vi "fpga_status.vi"(8 "error in (no error)":errorcluster, 11 "pulse_gen_and_detect_p2p in":refnum<class "pulse_gen_and_detect_p2p.lvclass">) -> (0 "error out":errorcluster, 2 "pulse TX status":T1, 3 "pulse_gen_and_detect_p2p out":refnum<class "pulse_gen_and_detect_p2p.lvclass">)   [LabVIEW 2021, in "pulse_gen_and_detect_p2p.lvclass"]
uses:
  pulse_gen_and_detect_p2p.lvclass
  pulse_gen_and_detect_p2p.lvclass/pulse_gen_and_detect_p2p.ctl
  fpga/vis/pulse detector/PDW interpoter params.ctl
  <vilib>/Utility/error.llb/Error Cluster From Error Code.vi
  <vilib>/rvi/errors/niLvFpgaAdjustHostInterfaceError.vi
  <vilib>/rvi/interface/nirviReadWriteControl/nirviReadWriteControl.xnode
  <vilib>/rvi/interface/nirviMethod/nirviMethod.xnode
  <resource>/objmgr/PeerToPeerStream.rc
  <vilib>/FPGAPlugInAG/Dynamic/niLvFpga_ReadFifo_Dynamic.vi
  <vilib>/rvi/errors/niLvFpgaMergeErrorWithErrorCode.vi
  NiFpgaLv.dll
  <vilib>/rvi/interface/Simulation/niFpgaSimulationCallBeginRW.vi
panel:
  out "tend":dbl
  out "amp":dbl
  out "pw":dbl
  out "f":dbl format="%_10e"
  out "num of Rx pulses":dbl
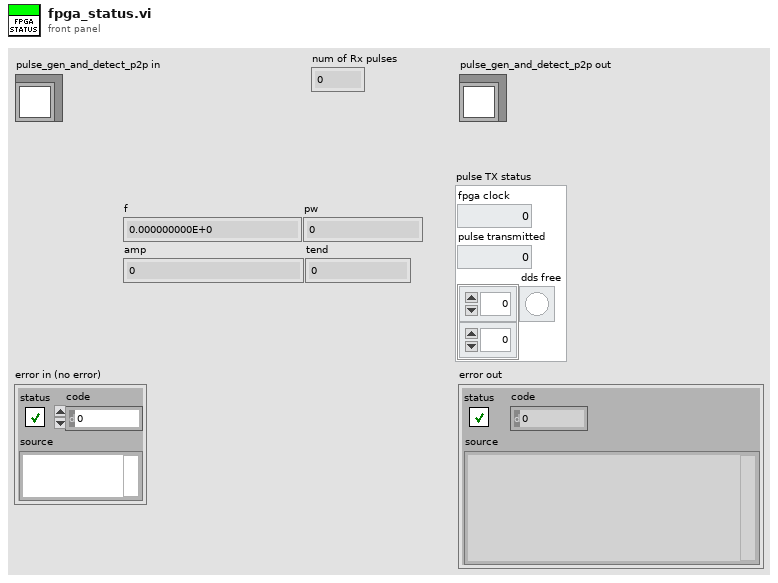
[diagram p1: front panel]
types:
  T1 = cluster{"fpga clock":dbl, "pulse transmitted":u32, "dds free":bool[][]}
  T2 = typedef "PDW interpoter params.ctl" = cluster{"Fs (Hz)":dbl, "fft size ":u32, "F base (Hz)":dbl, "min AMP (dB)":dbl, "PW low bar (fft cycle)":dbl, "Pw high bar (fft cycle)":dbl, "lo likege removal (fft bin)":i32, "max gap (fft cycle)":dbl}
  T3 = cluster{"fpga clock":u64, "pulse transmitted":u32, "dds free":bool[]}
  T4 = cluster{"min PW (fft cycels)":u16, "max PW (fft cycels)":u16, "max gap (fft cycels)":u8, "detection bar (liniar amp)":fxp<+,64,63>, "peak detect":bool}
  T5 = cluster{"f":dbl, "pw":dbl, "amp":dbl, "tend":dbl}[]
  T6 = cluster{"f":dbl, "pw":dbl, "amp":dbl, "tend":dbl}
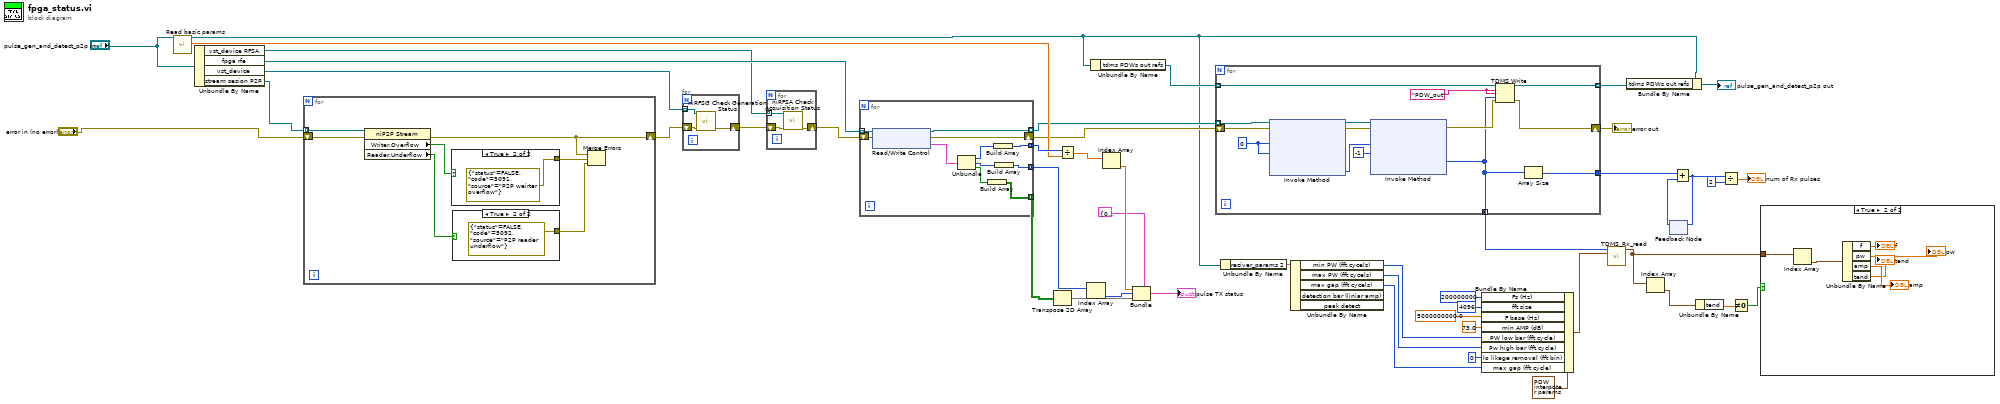
[diagram p0: block diagram]
diagram:
  n1 = call-dynamic "Read basic params.vi"("device_type in"="pulse_gen_and_detect_p2p in") -> ("device_type out"=w16:refnum<class "pulse_gen_and_detect_p2p.lvclass">, "Fs  FPGA"=w44:dbl)  [unwired: 13 in, 4 out]
  n2 = Unbundle By Name("pulse_gen_and_detect_p2p in") -> ("vst_device RFSA"=w29:refnum<k15>[], "fpga rfe"=w46:refnum<k20>[], "vst_device"=w37:refnum<k15>[], "stream sesion P2P"=w35:refnum<k20>[])
  n3 = for {
    shift-right: [w50] -> w36
    shift-left: "error in (no error)" -> [w54]
    tunnel: w35 -> [w53] mode=indexing
    n4 = property class="niP2P Stream"(reference=w53, error in=w54) -> (error out=w50:errorcluster, "Writer.Overflow"=w52:bool, "Reader.Underflow"=w51:bool)  [unwired: 1 out]
    n5 = case shown="True" w52 {
      tunnel: [_ errorcluster {"status"=FALSE, "code"=5091, "source"="P2P weirter overflow"} ("error out")] -> w49
      frame False {
      }
      frame True {
      }
    }
    n6 = case shown="True" w51 {
      tunnel: [_ errorcluster {"status"=FALSE, "code"=5092, "source"="P2P reader underflow"} ("error out")] -> w48
      frame False {
      }
      frame True {
      }
    }
    n7 = Merge Errors(w50, w49, w48) -> ()  [unwired: 1 out]
  }
  n8 = for {
    tunnel: w37 -> [w59] mode=indexing
    shift-right: [w57] -> w31
    shift-left: w36 -> [w58]
    n9 = call <instrlib>:"niRFSG Check Generation Status.vi"("instrument handle"=w59, "error in"=w58) -> ("error out"=w57:errorcluster)  [unwired: 11 in, 2 out]
  }
  n10 = for {
    tunnel: w29 -> [w60] mode=indexing
    shift-right: [w61] -> w30
    shift-left: w31 -> [w62]
    n11 = call <instrlib>:"niRFSA Check Acquisition Status.vi"("instrument handle"=w60, "error in"=w62) -> ("error out"=w61:errorcluster)  [unwired: 11 in, 2 out]
  }
  n12 = for {
    tunnel: w46 -> [w70] mode=indexing
    shift-right: [w72] -> w27
    shift-left: w30 -> [w73]
    tunnel: [w71] -> w28 mode=indexing
    tunnel: [w69] -> w45 mode=concatenating
    tunnel: [w68] -> w40 mode=concatenating
    tunnel: [w67] -> w47 mode=concatenating
    n13 = xnode "Read/Write Control"("FPGA VI Reference In"=w70, "error in"=w73) -> ("FPGA VI Reference Out"=w71:refnum<k20>, "error out"=w72:errorcluster, "pulse TX status"=w66:T3)
    n14 = Unbundle(w66) -> ("fpga clock"=w65:u64, "pulse transmitted"=w64:u32, "dds free"=w63:bool[])
    n15 = Build Array(w63) -> (w69:bool[][])
    n16 = Build Array(w65) -> (w67:u64[])
    n17 = Build Array(w64) -> (w68:u32[])
  }
  n18 = Transpose 2D Array(2D array=w45) -> (transposed array=w43:bool[][])
  n19 = Divide(x=w47, y=w44) -> (x/y=w42:dbl[])
  n20 = Index Array(array=w40) -> (element=w39:u32)  [unwired: 1 in]
  n21 = Unbundle By Name(w16) -> ("tdms PDWs out refs"=w24:refnum<k34>[])
  n22 = Index Array(array=w42) -> (element=w41:dbl)  [unwired: 1 in]
  n23 = Bundle(cluster=T1 {"fpga clock"=0.0, "pulse transmitted"=0, "dds free"=[[FALSE, FALSE, FALSE, FALSE, FALSE, FALSE, FALSE, FALSE, FALSE, FALSE, FALSE, FALSE, FALSE, FALSE, FALSE, FALSE]]} ("pulse TX status"), "fpga clock"=w41, "pulse transmitted"=w39, "dds free"=w43) -> (→"pulse TX status":T1)
  n24 = for {
    tunnel: w28 -> [w87] mode=indexing
    shift-right: [w77] -> w26
    shift-left: w27 -> [w86]
    tunnel: w24 -> [w80] mode=indexing
    tunnel: [w79] -> w23 mode=indexing
    tunnel: [w75] -> w22
    tunnel: [w74] -> w17 mode=concatenating
    w76 = "PDW_out" ("group name")
    w82 = u32 0 ("Number of Elements")
    n25 = xnode "Invoke Method"("FPGA VI Reference In"=w87, "error in"=w86, "Number of Elements"=w82, "Timeout (ms)"=w82) -> ("FPGA VI Reference Out"=w84:refnum<k20>, "error out"=w85:errorcluster, "Elements Remaining"=w83:u32)  [unwired: 1 out]
    n26 = xnode "Invoke Method"("FPGA VI Reference In"=w84, "error in"=w85, "Number of Elements"=w83, "Timeout (ms)"=-1) -> ("error out"=w78:errorcluster, "Data"=w74:u64[])  [unwired: 2 out]
    n27 = TDMS Write(0:w80, 5:w76, 7:w76, 9:w74, 11:w78) -> (4:w79:refnum<k34>, 15:w77:errorcluster)  [unwired: 1 in, 2 out]
    n28 = Array Size(array=w74) -> (size(s)=w75:i32)
  }
  "error out" <- w26
  n29 = Unbundle By Name(w16) -> ("reciver_params 2"=w15:T4)
  n30 = Unbundle By Name(w15) -> ("min PW (fft cycels)"=w9:u16, "max PW (fft cycels)"=w10:u16, "max gap (fft cycels)"=w11:u8)  [unwired: 2 out]
  n31 = Bundle By Name(cluster=T2 {"Fs (Hz)"=200000000.0, "fft size "=4096, "F base (Hz)"=2000000000.0, "min AMP (dB)"=0.0, "PW low bar (fft cycle)"=0.0, "Pw high bar (fft cycle)"=7000.0, "lo likege removal (fft bin)"=-1, "max gap (fft cycle)"=0.0} ("PDW interpoter params"), "Fs (Hz)"=u32 200000000, "fft size"=u32 4096, "F base (Hz)"=5000000000.0, "min AMP (dB)"=73.0, "PW low bar (fft cycle)"=w9, "Pw high bar (fft cycle)"=w10, "lo likege removal (fft bin)"=0, "max gap (fft cycle)"=w11) -> (w13:T2)
  n32 = call "TDMS_Rx_read.vi"("Array in"=w17, "PDW interpoter params"=w13) -> ("Array"=w4:T5)  [unwired: 11 in, 2 out]
  n33 = Bundle By Name(cluster=w16, "tdms PDWs out refs"=w23) -> (→"pulse_gen_and_detect_p2p out":refnum<class "pulse_gen_and_detect_p2p.lvclass">)
  n34 = Index Array(array=w4) -> (element=w5:T6)  [unwired: 1 in]
  n35 = feedback #1() -> (w21:i32)  [unwired: 1 in]
  n36 = Add(x=w22, y=w21) -> (x+y=w20:i32)
  n37 = feedback-in #1(w20) -> ()
  n38 = Unbundle By Name(w5) -> ("tend"=w3:dbl)
  n39 = Divide(x=w20, y=2) -> (x/y=→"num of Rx pulses":dbl)
  n40 = Not Equal To 0?(x=w3) -> (x != 0?=w2:bool)
  n41 = case shown="True" w2 {
    tunnel: w4 -> [_ w88]
    frame False {
    }
    frame True {
      n42 = Index Array(array=w88) -> (element=w93:T6)  [unwired: 1 in]
      n43 = Unbundle By Name(w93) -> ("f"=→"f":dbl, "pw"=→"pw":dbl, "amp"=→"amp":dbl, "tend"=→"tend":dbl)
    }
  }
